vi "SenderUI.vi"(0 "Data Type":string(combo), 5 "Send":bool, 7 "Transmission Type":T1, 9 "Stop Stream":bool, 11 "error in (no error)":errorcluster) -> (15 "error out":errorcluster)   [LabVIEW 2023, in "Sender.lvclass"]
doc: "This SenderUI Vi allows the user to choose the data type of the data that is being sent to the receiver along with the transmission type like with data, without data and stream data."
uses:
  Sender.lvclass
  TypeDefs/TransmissionType.ctl
  TypeDefs/SenderQueueOperations.ctl
  TypeDefs/SenderStateDataCluster.ctl
  TypeDefs/SenderDataType.ctl
  TypeDefs/UserEventOperations.ctl
  TypeDefs/UserEventDataCluster.ctl
  Communication/Communication.lvclass
  TypeDefs/ReceiverQueueOperations.ctl
  TypeDefs/ReceiverStateDataCluster.ctl
  Receiver/ReceiverUI.vi
  Sender.lvclass/Sender.ctl
  Receiver/Receiver.lvclass
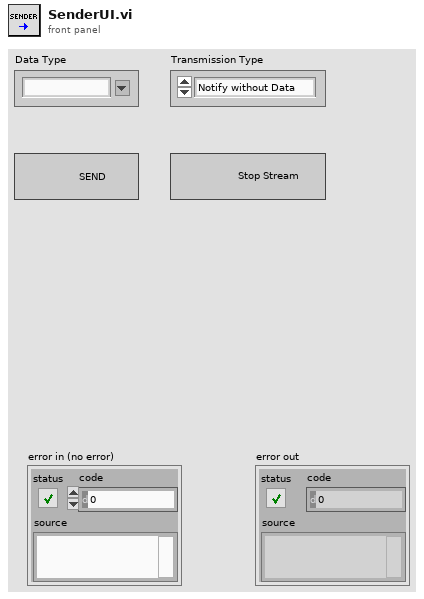
[diagram p1: front panel]
types:
  T1 = typedef "TransmissionType.ctl" = enum16{"Notify without Data", "Notify with Data", "Stream Data"}
  T2 = typedef "UserEventDataCluster.ctl" = cluster{"State":string, "Data":variant}
  T3 = typedef "UserEventOperations.ctl" = enum16{"Create", "Generate", "Release"}
  T4 = typedef "SenderDataType.ctl" = cluster{"DataType":string, "Send":bool, "Class Base Path":path, "Sender class":refnum<class "Sender.lvclass">, "Data Type Path":path, "Transmission Type":T1, "Start Time":dbl, "Stop Stream":bool, "Start Com":bool, "TCP connection ID":refnum<k5>}
  T5 = typedef "SenderQueueOperations.ctl" = enum16{"Create", "Enqueue", "Dequeue", "Enqueue N", "Flush", "Close", "Enqueue N Stack"}
  T6 = typedef "SenderStateDataCluster.ctl" = cluster{"State":string, "Data":variant}
  T7 = typedef "ReceiverStateDataCluster.ctl" = cluster{"State":string, "Data":variant}
  T8 = typedef "ReceiverQueueOperations.ctl" = enum16{"Create", "Enqueue", "Dequeue", "Enqueue N", "Flush", "Close", "Enqueue N Stack"}
  T9 = enum8{"Enabled", "Disabled", "Disabled and Grayed Out"}
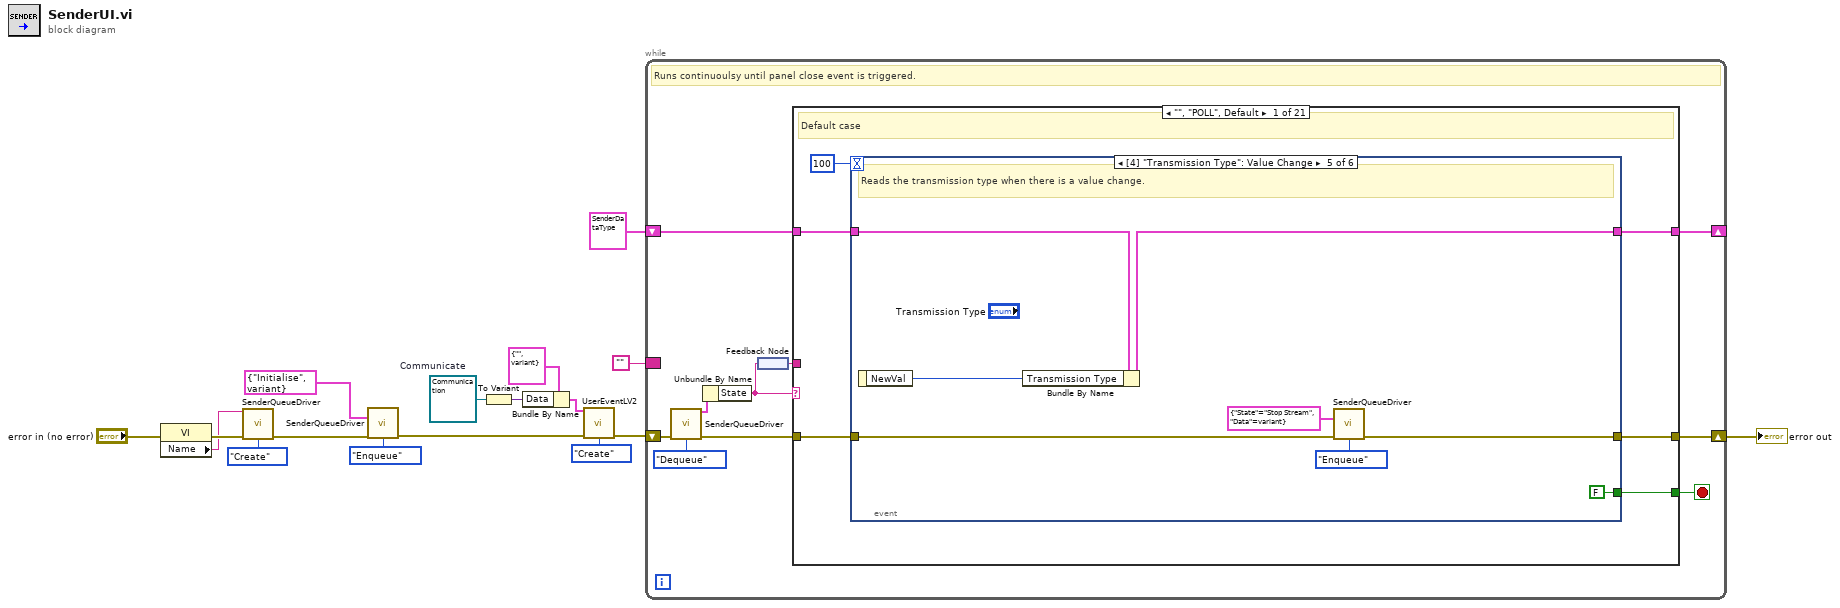
[diagram p0: block diagram]
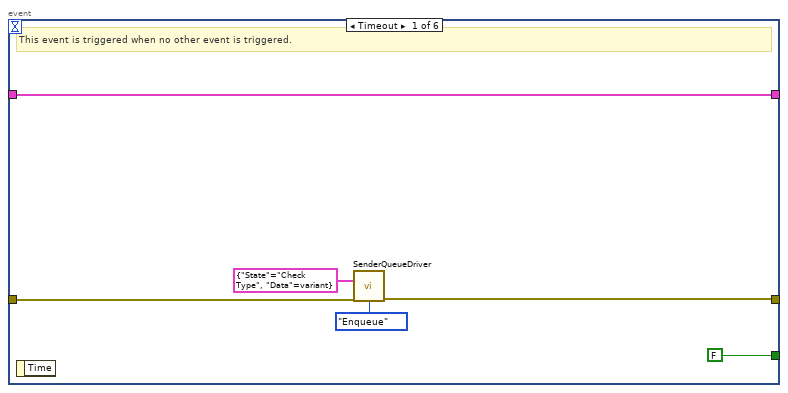
[diagram p2: hidden frame]
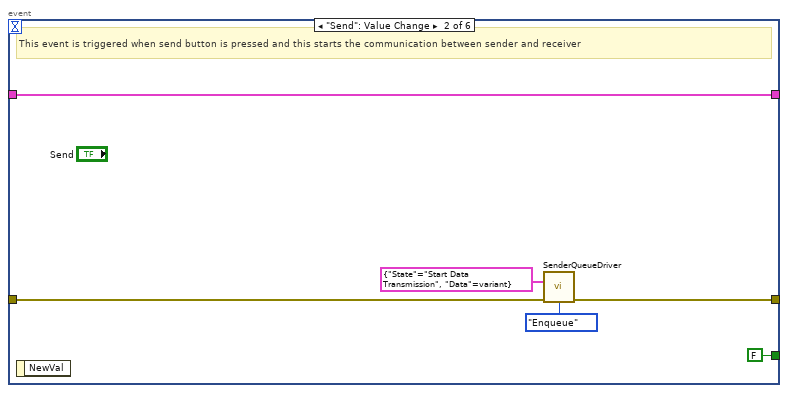
[diagram p3: hidden frame]
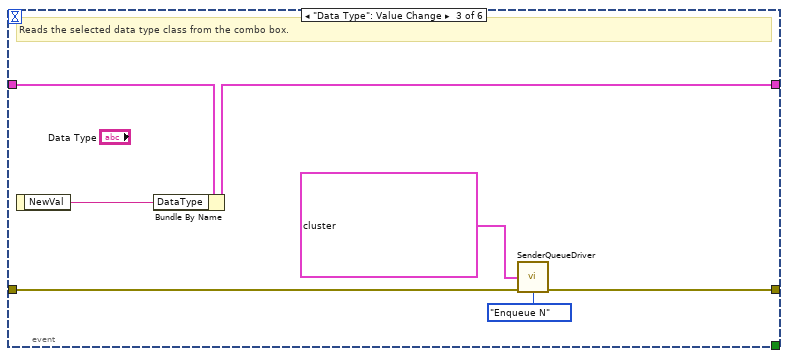
[diagram p4: hidden frame]
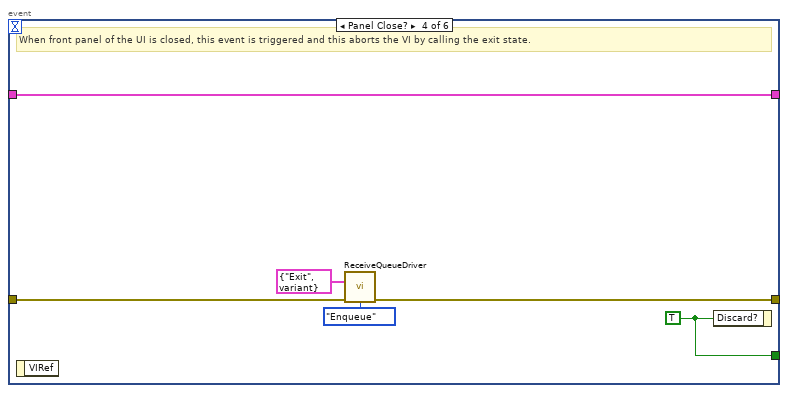
[diagram p5: hidden frame]
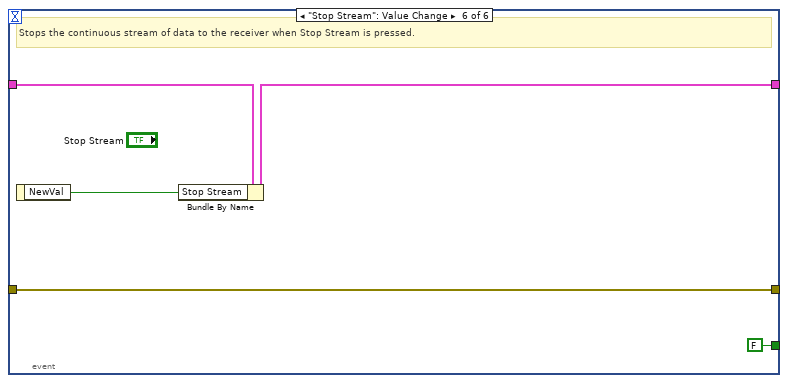
[diagram p6: hidden frame]
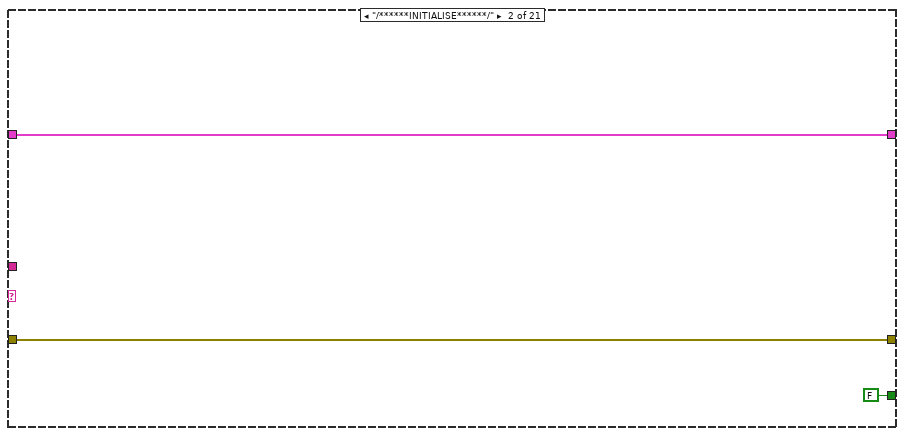
[diagram p7: hidden frame]
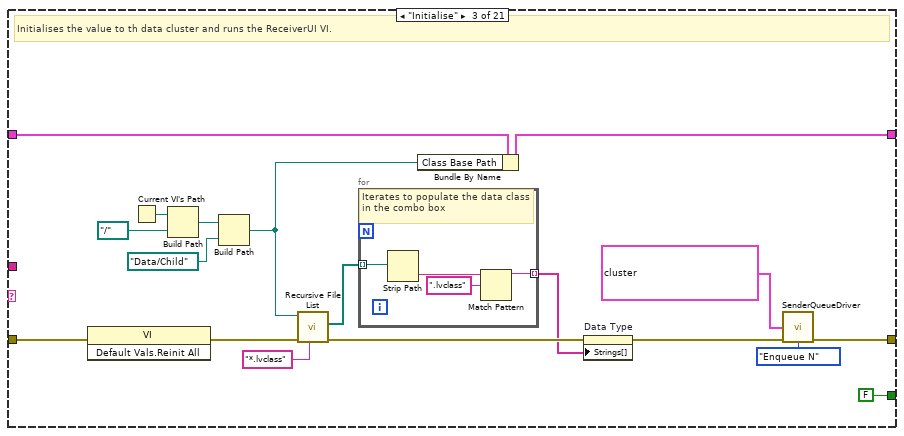
[diagram p8: hidden frame]
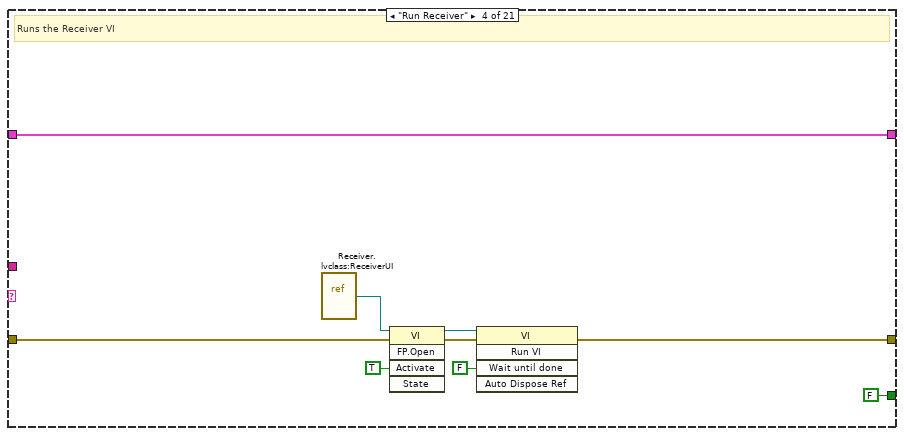
[diagram p9: hidden frame]
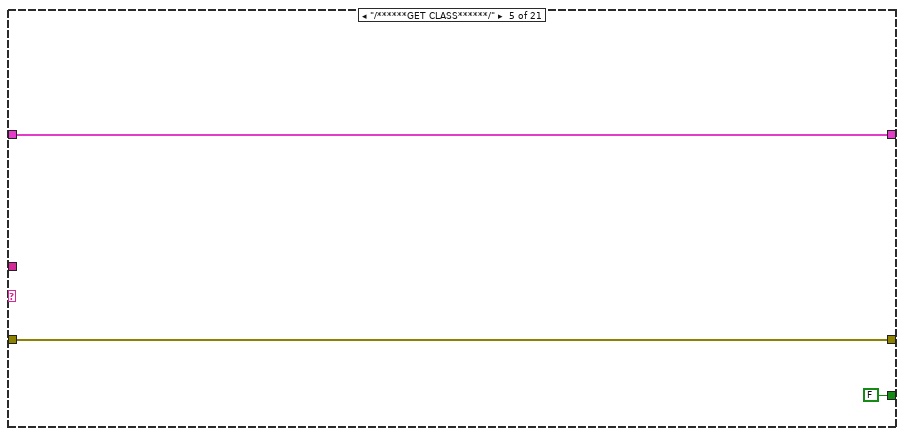
[diagram p10: hidden frame]
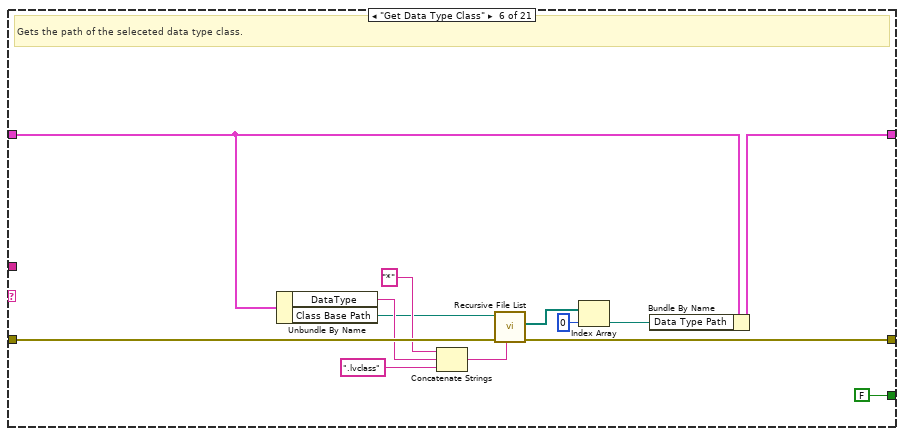
[diagram p11: hidden frame]
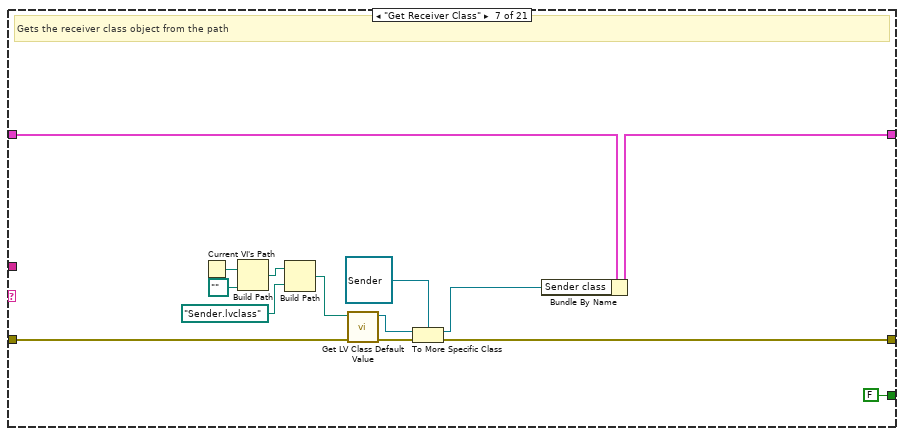
[diagram p12: hidden frame]
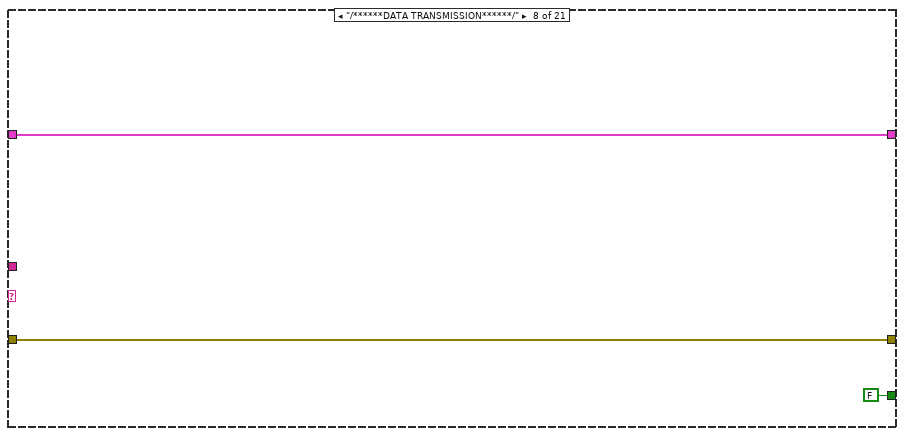
[diagram p13: hidden frame]
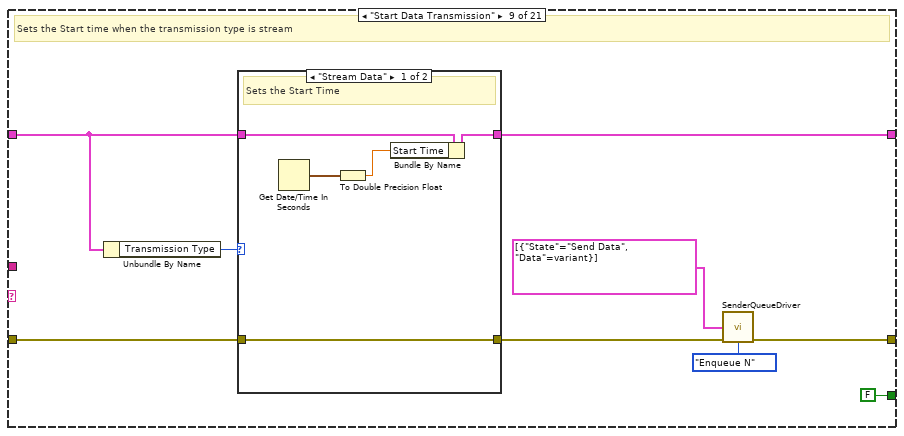
[diagram p14: hidden frame]
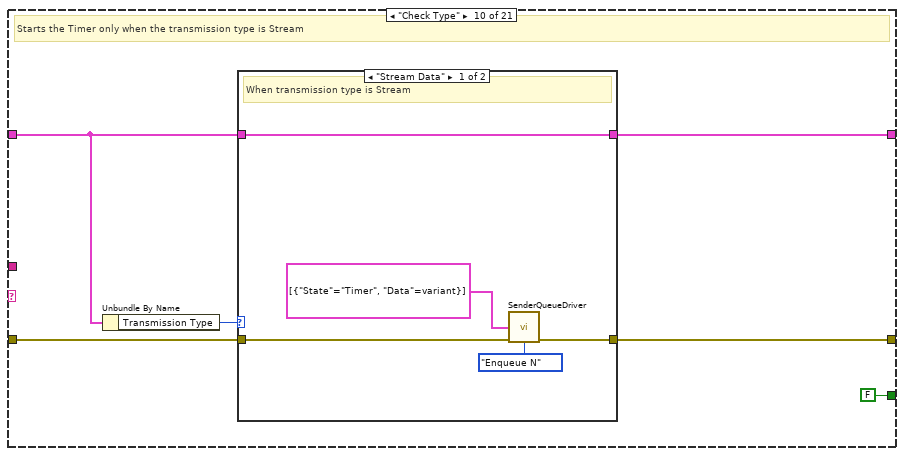
[diagram p16: hidden frame]
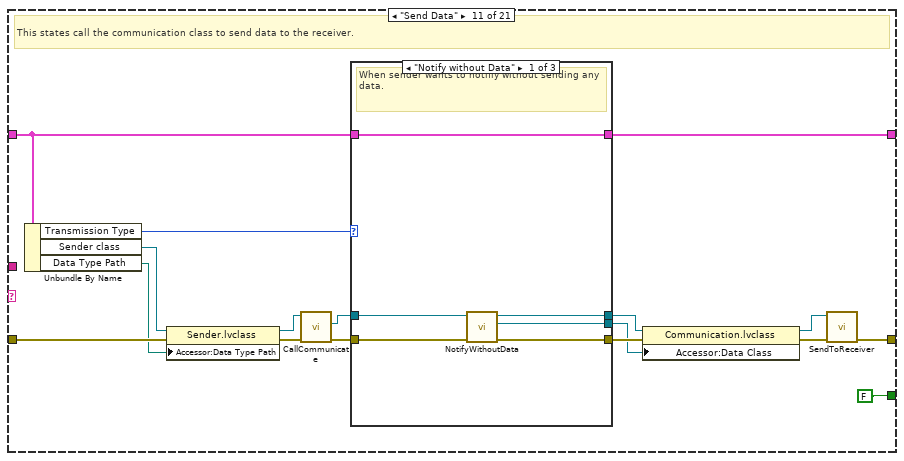
[diagram p18: hidden frame]
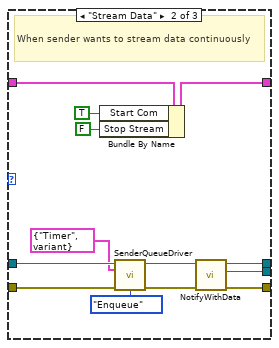
[diagram p19: hidden frame]
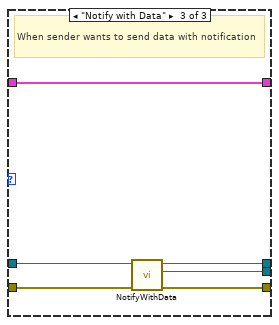
[diagram p20: hidden frame]
diagram:
  w4 = refnum<class "Communication.lvclass"> refnum  # Communicate
  n1 = property class="VI"(error in="error in (no error)") -> (error out=w2:errorcluster, "Name"=w1:string)  [unwired: 1 in, 1 out]
  n2 = call "SenderQueueDriver.vi"("Queue Name"=w1, "error in (no error)"=w2, "Enum"=SenderQueueOperations."Create") -> ("error out"=w15:errorcluster)  [unwired: 11 in, 1 out]
  n3 = call "SenderQueueDriver.vi"("Enqueue Element"=T6 {"State"="Initialise", "Data"=variant}, "error in (no error)"=w15, "Enum"=SenderQueueOperations."Enqueue") -> ("error out"=w9:errorcluster)  [unwired: 11 in, 1 out]
  n4 = To Variant(anything=w4) -> (Variant=w3:variant)
  n5 = Bundle By Name(cluster=T2 {"State"="", "Data"=variant} ("Data"), "Data"=w3) -> (w5:T2)
  n6 = call "UserEventLV2.vi"("Data"=w5, "Error In"=w9, "Operation"=UserEventOperations."Create") -> ("Error Out"=w8:errorcluster)  [unwired: 11 in, 1 out]
  n7 = while {
    shift-right: [w27] -> w17
    shift-left: w8 -> [w26]
    shift-right: [w18] -> _
    shift-left: T4 {"DataType"="", "Send"=FALSE, "Class Base Path"=path "", "Sender class"=refnum, "Data Type Path"=path "", "Transmission Type"=enum."Notify without Data", "Start Time"=0.0, "Stop Stream"=FALSE, "Start Com"=FALSE, "TCP connection ID"=refnum} -> [w19]
    border: "" -> [_]
    stop <- w23 stop-if-true
    # "Runs continuoulsy until panel close event is triggered."
    n8 = call "SenderQueueDriver.vi"("error in (no error)"=w26, "Enum"=SenderQueueOperations."Dequeue") -> ("Dequeue Element"=w24:T6, "error out"=w25:errorcluster)  [unwired: 12 in]
    n9 = Unbundle By Name(w24) -> ("State"=w21:string)
    n10 = feedback-in #1(w21) -> ()
    n11 = feedback #1() -> (w20:string)
    n12 = case shown="\"\", \"POLL\", Default" w21 {
      tunnel: w25 -> [w32 w73 w85 w100 w107 w119 w126 w137 w147 w160 w184 w210 w217 w249 w252 w265 w278 w282 w287 w291 w294]
      tunnel: [w31 w73 w76 w99 w107 w109 w125 w137 w140 w155 w168 w210 w216 w249 w252 w255 w278 w281 w286 w291 w296] -> w27
      tunnel: [w33 FALSE ("Discard?") FALSE FALSE ("Discard?") FALSE ("Discard?") FALSE ("Discard?") FALSE ("Discard?") FALSE ("Discard?") FALSE ("Discard?") FALSE ("Discard?") FALSE FALSE ("Discard?") FALSE ("Discard?") FALSE ("Discard?") FALSE ("Discard?") FALSE ("Discard?") FALSE ("Discard?") FALSE ("Discard?") FALSE ("Discard?") FALSE ("Discard?") TRUE] -> w23
      tunnel: w20 -> [_ _ _ _ _ _ _ _ _ _ _ _ _ _ _ w263 _ _ _ _ _]
      tunnel: w19 -> [w29 w74 w83 w98 w108 w120 w127 w138 w144 w157 w172 w211 w215 w250 w253 w268 w279 w284 w289 w292 w301]
      tunnel: [w28 w74 w80 w98 w108 w112 w123 w138 w143 w156 w171 w211 w214 w247 w253 w268 w279 w284 w289 w292 w301] -> w18
      frame "", "POLL", Default {
        # "Default case"
        n13 = event shown="[4] \"Transmission Type\": Value Change" {
          selector: _ -> [_ _ _ _ _ _]
          dyn-events: _ -> [_ _ _ _ _ _]
          timeout: 100 -> [_ _ _ _ _ _]
          tunnel: [FALSE FALSE _ w57 FALSE ("Discard?") FALSE ("Discard?")] -> w33
          tunnel: w32 -> [w36 w42 w47 w55 w60 w67]
          tunnel: [w35 w41 w48 w54 w59 w67] -> w31
          tunnel: w29 -> [w38 w45 w52 w58 w66 w71]
          tunnel: [w38 w45 w51 w58 w65 w69] -> w28
          event Timeout {
            # "This event is triggered when no other event is triggered."
            n14 = event-data() -> ()  [unwired: 1 in, 1 out]
            n15 = call "SenderQueueDriver.vi"("Enqueue Element"=T6 {"State"="Check Type", "Data"=variant}, "error in (no error)"=w36, "Enum"=SenderQueueOperations."Enqueue") -> ("error out"=w35:errorcluster)  [unwired: 11 in, 1 out]
          }
          event "Send": Value Change {
            # "This event is triggered when send button is pressed and this starts the communication between sender and receiver"
            n16 = event-data() -> ()  [unwired: 1 in, 1 out]
            n17 = call "SenderQueueDriver.vi"("Enqueue Element"=T6 {"State"="Start Data Transmission", "Data"=variant}, "error in (no error)"=w42, "Enum"=SenderQueueOperations."Enqueue") -> ("error out"=w41:errorcluster)  [unwired: 11 in, 1 out]
          }
          event "Data Type": Value Change {
            # "Reads the selected data type class from the combo box."
            n18 = event-data() -> ("NewVal"=w50:string)  [unwired: 1 in]
            n19 = Bundle By Name(cluster=w52, "DataType"=w50) -> (w51:T4)
            n20 = call "SenderQueueDriver.vi"("Enqueue N Element"=T6[] [{"State"="Get Data Type Class", "Data"=variant}, {"State"="Enable Controls", "Data"=variant}, {"State"="Get Receiver Class", "Data"=variant}], "error in (no error)"=w47, "Enum"=SenderQueueOperations."Enqueue N") -> ("error out"=w48:errorcluster)  [unwired: 11 in, 1 out]
          }
          event Panel Close? {
            w57 = TRUE ("Discard?")
            # "When front panel of the UI is closed, this event is triggered and this aborts the VI by calling the exit state."
            n21 = event-data() -> ()  [unwired: 1 in, 1 out]
            n22 = call "ReceiveQueueDriver.vi"("Enqueue Element"=T7 {"State"="Exit", "Data"=variant}, "error in (no error)"=w55, "Enum"=ReceiverQueueOperations."Enqueue") -> ("error out"=w54:errorcluster)  [unwired: 11 in, 1 out]
            n23 = event-data("Discard?"=w57) -> ()  [unwired: 1 in, 1 out]
          }
          event Value Change {
            # "Reads the transmission type when there is a value change."
            n24 = event-data() -> ("NewVal"=w64:T1)  [unwired: 1 in]
            n25 = Bundle By Name(cluster=w66, "Transmission Type"=w64) -> (w65:T4)
            n26 = call "SenderQueueDriver.vi"("Enqueue Element"=T6 {"State"="Stop Stream", "Data"=variant}, "error in (no error)"=w60, "Enum"=SenderQueueOperations."Enqueue") -> ("error out"=w59:errorcluster)  [unwired: 11 in, 1 out]
          }
          event "Stop Stream": Value Change {
            # "Stops the continuous stream of data to the receiver when Stop Stream is pressed."
            n27 = event-data() -> ("NewVal"=w68:bool)  [unwired: 1 in]
            n28 = Bundle By Name(cluster=w71, "Stop Stream"=w68) -> (w69:T4)
          }
        }
      }
      frame "/******INITIALISE******/" {
      }
      frame "Initialise" {
        # "Initialises the value to th data cluster and runs the ReceiverUI VI."
        n29 = invoke class="VI" method="Default Vals.Reinit All"(error in=w85) -> (error out=w82:errorcluster)  [unwired: 2 in, 2 out]
        n30 = Current VI's Path() -> (path=w88:path)
        n31 = Build Path(base path=w88, name or relative path=path "../..") -> (appended path=w87:path)
        n32 = Build Path(base path=w87, name or relative path=path "Data/Child") -> (appended path=w79:path)
        n33 = call <vilib>:"Recursive File List.vi"("pattern"="*.lvclass", "error in (no error)"=w82, "Folder Path"=w79) -> ("error out"=w84:errorcluster, "All Files in Dir"=w89:path[])  [unwired: 4 in, 3 out]
        n34 = for {
          tunnel: w89 -> [w96] mode=indexing
          tunnel: [w93] -> w81 mode=indexing
          # "Iterates to populate the data class in the combo box"
          n35 = Strip Path(path=w96) -> (name=w95:string)  [unwired: 1 out]
          n36 = Match Pattern(string=w95, regular expression=".lvclass") -> (before substring=w93:string)  [unwired: 1 in, 3 out]
        }
        n37 = Bundle By Name(cluster=w83, "Class Base Path"=w79) -> (w80:T4)
        n38 = property on="Data Type" class="CmbBox"(error in=w84, "Strings[]"=w81) -> (error out=w78:errorcluster)  [unwired: 1 in, 1 out]
        n39 = call "SenderQueueDriver.vi"("Enqueue N Element"=T6[] [{"State"="Run Receiver", "Data"=variant}, {"State"="Disable Controls", "Data"=variant}], "error in (no error)"=w78, "Enum"=SenderQueueOperations."Enqueue N") -> ("error out"=w76:errorcluster)  [unwired: 11 in, 1 out]
      }
      frame "Run Receiver" {
        # "Runs the Receiver VI"
        n40 = vi-ref "Receiver.lvclass:ReceiverUI.vi"() -> (w104:refnum<vi>)
        n41 = invoke class="VI" method="FP.Open"(reference=w104, error in=w100, "Activate"=TRUE ("Activate?")) -> (reference out=w102:refnum<vi>, error out=w103:errorcluster)  [unwired: 2 in, 3 out]
        n42 = invoke class="VI" method="Run VI"(reference=w102, error in=w103, "Wait until done"=FALSE ("Wait Until Done")) -> (error out=w99:errorcluster)  [unwired: 2 in, 4 out]
      }
      frame "/******GET CLASS******/" {
      }
      frame "Get Data Type Class" {
        # "Gets the path of the seleceted data type class."
        n43 = Unbundle By Name(w120) -> ("DataType"=w117:string, "Class Base Path"=w110:path)
        n44 = Concatenate Strings("*" ("string"), w117, ".lvclass" ("pattern")) -> (w115:string)
        n45 = call <vilib>:"Recursive File List.vi"("pattern"=w115, "error in (no error)"=w119, "Folder Path"=w110) -> ("error out"=w109:errorcluster, "All Files in Dir"=w114:path[])  [unwired: 4 in, 3 out]
        n46 = Index Array(array=w114, index=0) -> (element=w111:path)
        n47 = Bundle By Name(cluster=w120, "Data Type Path"=w111) -> (w112:T4)
      }
      frame "Get Receiver Class" {
        # "Gets the receiver class object from the path"
        n48 = Current VI's Path() -> (path=w135:path)
        n49 = Build Path(base path=w135, name or relative path=path "..") -> (appended path=w133:path)
        n50 = Build Path(base path=w133, name or relative path=path "Sender.lvclass") -> (appended path=w131:path)
        n51 = call <vilib>:"Get LV Class Default Value.vi"("error in (no error)"=w126, "class path"=w131) -> ("error out"=w130:errorcluster, "object"=w129:refnum<class>)  [unwired: 8 in]
        n52 = To More Specific Class(target class=refnum<class "Sender.lvclass"> refnum ("Sender.lvclass"), reference=w129, error in=w130) -> (specific class reference=w122:refnum<class "Sender.lvclass">, error out=w125:errorcluster)
        n53 = Bundle By Name(cluster=w127, "Sender class"=w122) -> (w123:T4)
      }
      frame "/******DATA TRANSMISSION******/" {
      }
      frame "Start Data Transmission" {
        # "Sets the Start time when the transmission type is stream"
        n54 = Unbundle By Name(w144) -> ("Transmission Type"=w145:T1)
        n55 = case shown="\"Stream Data\"" w145 {
          tunnel: w147 -> [w148 w153]
          tunnel: [w148 w153] -> w141
          tunnel: w144 -> [w152 w154]
          tunnel: [w151 w154] -> w143
          frame "Stream Data" {
            # "Sets the Start Time"
            n56 = Get Date/Time In Seconds() -> (seconds since 1Jan1904=w150:timestamp)
            n57 = To Double Precision Float(number=w150) -> (double precision float=w149:dbl)
            n58 = Bundle By Name(cluster=w152, "Start Time"=w149) -> (w151:T4)
          }
          frame Default {
            # "Default"
          }
        }
        n59 = call "SenderQueueDriver.vi"("Enqueue N Element"=T6[] [{"State"="Send Data", "Data"=variant}], "error in (no error)"=w141, "Enum"=SenderQueueOperations."Enqueue N") -> ("error out"=w140:errorcluster)  [unwired: 11 in, 1 out]
      }
      frame "Check Type" {
        # "Starts the Timer only when the transmission type is Stream"
        n60 = Unbundle By Name(w157) -> ("Transmission Type"=w158:T1)
        n61 = case shown="\"Stream Data\"" w158 {
          tunnel: w160 -> [w164 w166]
          tunnel: [w163 w166] -> w155
          tunnel: w157 -> [w161 w167]
          tunnel: [w161 w167] -> w156
          frame "Stream Data" {
            # "When transmission type is Stream"
            n62 = call "SenderQueueDriver.vi"("Enqueue N Element"=T6[] [{"State"="Timer", "Data"=variant}], "error in (no error)"=w164, "Enum"=SenderQueueOperations."Enqueue N") -> ("error out"=w163:errorcluster)  [unwired: 11 in, 1 out]
          }
          frame Default {
            # "Default"
          }
        }
      }
      frame "Send Data" {
        # "This states call the communication class to send data to the receiver."
        n63 = Unbundle By Name(w172) -> ("Transmission Type"=w173:T1, "Sender class"=w175:refnum<class "Sender.lvclass">, "Data Type Path"=w174:path)
        n64 = property class="Sender.lvclass"(reference=w175, error in=w184, "Accessor:Data Type Path"=w174) -> (reference out=w176:refnum<class "Sender.lvclass">, error out=w177:errorcluster)
        n65 = call "CallCommunicate.vi"("error in (no error)"=w177, "Sender in"=w176) -> ("error out"=w183:errorcluster, "Communication.lvclass"=w178:refnum<class "Communication.lvclass">)  [unwired: 7 in, 1 out]
        n66 = case shown="\"Notify without Data\"" w173 {
          tunnel: w183 -> [w190 w198 w208]
          tunnel: [w189 w201 w207] -> w182
          tunnel: [w186 w199 w206] -> w181
          tunnel: [w187 w200 w205] -> w180
          tunnel: w178 -> [w188 w202 w204]
          tunnel: w172 -> [w185 w192 w203]
          tunnel: [w185 w191 w203] -> w171
          frame "Notify without Data" {
            # "When sender wants to notifiy without sending any data."
            n67 = call "NotifyWithoutData.vi"("error in (no error)"=w190, "Communication in"=w188) -> ("error out"=w189:errorcluster, "Data out"=w187:refnum<class "Data.lvclass">, "Communication out"=w186:refnum<class "Communication.lvclass">)  [unwired: 7 in]
          }
          frame "Stream Data" {
            # "When sender wants to stream data continuously"
            n68 = Bundle By Name(cluster=w192, "Start Com"=TRUE, "Stop Stream"=FALSE) -> (w191:T4)
            n69 = call "SenderQueueDriver.vi"("Enqueue Element"=T6 {"State"="Timer", "Data"=variant}, "error in (no error)"=w198, "Enum"=SenderQueueOperations."Enqueue") -> ("error out"=w197:errorcluster)  [unwired: 11 in, 1 out]
            n70 = call "NotifyWithData.vi"("error in (no error)"=w197, "Communication in"=w202) -> ("error out"=w201:errorcluster, "Data out"=w200:refnum<class "Data.lvclass">, "Communication out"=w199:refnum<class "Communication.lvclass">)  [unwired: 7 in]
          }
          frame "Notify with Data" {
            # "When sender wants to send data with notification"
            n71 = call "NotifyWithData.vi"("error in (no error)"=w208, "Communication in"=w204) -> ("error out"=w207:errorcluster, "Data out"=w205:refnum<class "Data.lvclass">, "Communication out"=w206:refnum<class "Communication.lvclass">)  [unwired: 7 in]
          }
        }
        n72 = property class="Communication.lvclass"(reference=w181, error in=w182, "Accessor:Data Class"=w180) -> (reference out=w170:refnum<class "Communication.lvclass">, error out=w169:errorcluster)
        n73 = call "SendToReceiver.vi"("error in (no error)"=w169, "Communication in"=w170) -> ("error out"=w168:errorcluster)  [unwired: 8 in, 1 out]
      }
      frame "/*****TIMER******/" {
      }
      frame "Timer" {
        # "Runs the timer for Stream data transmission type."
        n74 = Unbundle By Name(w215) -> ("Start Time"=w218:dbl, "Start Com"=w213:bool, "Stop Stream"=w212:bool)
        n75 = case shown="True" w213 {
          tunnel: w218 -> [_ w232]
          tunnel: w217 -> [w220 w231]
          tunnel: [w220 w230] -> w216
          tunnel: w215 -> [w221 w229]
          tunnel: [w221 w228] -> w214
          tunnel: w212 -> [_ w222]
          frame False {
            # "When Start communication boolean is false, timer won't run"
          }
          frame True {
            # "When Start communication boolean is true, timer runs"
            n76 = Get Date/Time In Seconds() -> (seconds since 1Jan1904=w227:timestamp)
            n77 = To Double Precision Float(number=w227) -> (double precision float=w223:dbl)
            n78 = Subtract(x=w223, y=w232) -> (x-y=w226:dbl)
            n79 = Greater Or Equal?(x=w226, y=1.0) -> (x >= y?=w224:bool)
            n80 = case shown="True" w224 {
              tunnel: w231 -> [w238 w244]
              tunnel: [w237 w244] -> w230
              tunnel: w229 -> [w242 w243]
              tunnel: [w241 w243] -> w228
              tunnel: w223 -> [w240 _]
              tunnel: w222 -> [w236 _]
              frame True {
                # "When elapsed time is >= 1, timer is resetted and data is sent to the receiver."
                n81 = Bundle By Name(cluster=w242, "Start Time"=w240) -> (w241:T4)
                n82 = Select(t=T6[] [{"State"="Stop Stream", "Data"=variant}] ("f"), s=w236, f=T6[] [{"State"="Send Data", "Data"=variant}]) -> (s? t:f=w233:T6[])
                n83 = call "SenderQueueDriver.vi"("Enqueue N Element"=w233, "error in (no error)"=w238, "Enum"=SenderQueueOperations."Enqueue N") -> ("error out"=w237:errorcluster)  [unwired: 11 in, 1 out]
              }
              frame False {
                # "When elapsed time is < 1, timer continuous to run"
              }
            }
          }
        }
      }
      frame "Stop Stream" {
        # "When Stop Stream button is pressed, this state is called, timer is stopped and data communication is also stopped."
        n84 = Bundle By Name(cluster=w250, "Start Time"=0.0, "Start Com"=FALSE) -> (w247:T4)
      }
      frame "/******ERROR******/" {
      }
      frame "Error" {
        # "This state is called when any occurs."
        n85 = Unbundle By Name(w265) -> ("status"=w262:bool, "code"=w261:i32)
        n86 = call <vilib>:"Clear Errors.vi"("error in (no error)"=w265) -> ("error out"=w266:errorcluster)  [unwired: 5 in, 1 out]
        n87 = Format Into String(format string="Erro Occured at state : %s \nErro Status : %s \nError Code : %d", initial string="", error in=w266, w263, w262, w261) -> (resulting string=w259:string, error out=w256:errorcluster)
        n88 = Two Button Dialog(message=w259, 1:"Exit" ("F button name (\"Cancel\")"), 2:"Continue" ("T button name (\"OK\")")) -> (T button?=w254:bool)
        n89 = case shown="False" w254 {
          tunnel: w256 -> [w269 w275]
          tunnel: [w269 w272] -> w255
          frame True {
            # "when user continues"
          }
          frame False {
            # "When user exits after an error"
            n90 = call "SenderQueueDriver.vi"("Enqueue Element"=T6 {"State"="Exit", "Data"=variant}, "error in (no error)"=w275, "Enum"=SenderQueueOperations."Enqueue") -> ("error out"=w273:errorcluster)  [unwired: 11 in, 1 out]
            n91 = call "ReceiveQueueDriver.vi"("Enqueue Element"=T7 {"State"="Exit", "Data"=variant}, "error in (no error)"=w273, "Enum"=ReceiverQueueOperations."Enqueue") -> ("error out"=w272:errorcluster)  [unwired: 11 in, 1 out]
          }
        }
      }
      frame "/******FRONT PANEL ENABLE DISABLE******/" {
      }
      frame "Enable Controls" {
        # "Enables the control"
        n92 = property on="Send" class="Bool"(error in=w282, "DisabledEnum"=T9."Enabled" ("Disabled")) -> (error out=w281:errorcluster)  [unwired: 1 in, 1 out]
      }
      frame "Disable Controls" {
        # "Disables the control"
        n93 = property on="Send" class="Bool"(error in=w287, "DisabledEnum"=T9."Disabled and Grayed Out" ("Disabled")) -> (error out=w286:errorcluster)  [unwired: 1 in, 1 out]
      }
      frame "/******EXIT******/" {
      }
      frame "Exit" {
        # "Exits this sender VI."
        n94 = call "UserEventLV2.vi"("Error In"=w294, "Operation"=UserEventOperations."Release") -> ("Error Out"=w293:errorcluster)  [unwired: 12 in, 1 out]
        n95 = call "SenderQueueDriver.vi"("error in (no error)"=w293, "Enum"=SenderQueueOperations."Flush") -> ("error out"=w297:errorcluster)  [unwired: 12 in, 1 out]
        n96 = call "SenderQueueDriver.vi"("error in (no error)"=w297, "Enum"=SenderQueueOperations."Close") -> ("error out"=w296:errorcluster)  [unwired: 12 in, 1 out]
      }
    }
  }
  "error out" <- w17
